vi "lv-setBuildSpecTag.vi"(8 "error in (no error)":errorcluster, 9 "Tag value":string, 10 "Tag name":string, 11 "Project refs":T1={"LabVIEW Project Path"=path "C:/Users/admin/Desktop/Source/Waveform-Processing-Custom-Device.lvproj", "Project refnum"=refnum, "Build spec refnum"=refnum}) -> (0 "error out":errorcluster, 3 "Project refs out":T1={"LabVIEW Project Path"=path "C:/Users/admin/Desktop/Source/Waveform-Processing-Custom-Device.lvproj", "Project refnum"=refnum, "Build spec refnum"=refnum})   [LabVIEW 2014, in "lv-build-library.lvlib"]
uses:
  lv-build-library.lvlib
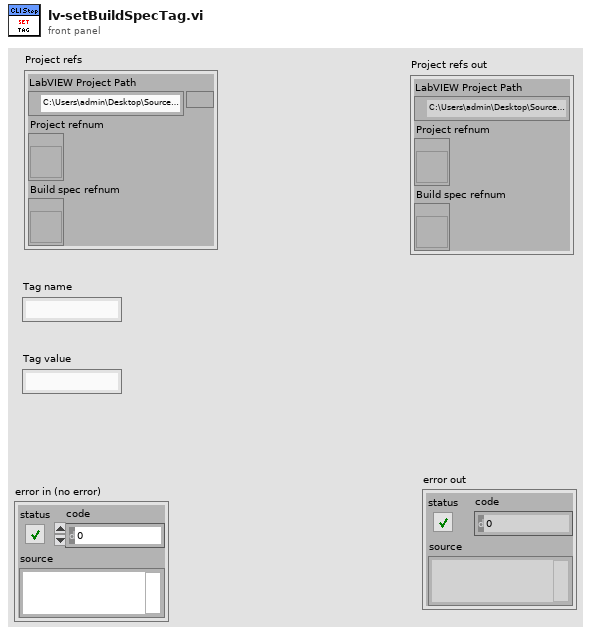
[diagram p1: front panel]
types:
  T1 = cluster{"LabVIEW Project Path":path, "Project refnum":refnum<vi>, "Build spec refnum":refnum<vi>}
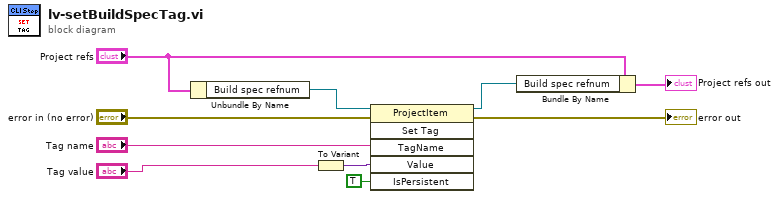
[diagram p0: block diagram]
diagram:
  n1 = Unbundle By Name("Project refs") -> ("Build spec refnum"=w4:refnum<vi>)
  n2 = To Variant(anything="Tag value") -> (Variant=w8:variant)
  n3 = invoke class="ProjectItem" method="Set Tag"(reference=w4, error in="error in (no error)", "TagName"="Tag name", "Value"=w8, "IsPersistent"=TRUE ("Is Persistent")) -> (reference out=w2:refnum<vi>, error out=→"error out":errorcluster)  [unwired: 1 in, 4 out]
  n4 = Bundle By Name(cluster="Project refs", "Build spec refnum"=w2) -> (→"Project refs out":T1)
